vi "Logging Message Loop.vi"(8 "error in (no error)":errorcluster, 10 "Data Queue":refnum<queue>, 11 "Message Queues":T1) -> (0 "error out":errorcluster)   [LabVIEW 2016, in "Logging.lvlib"]
doc: "The message loop subVI to handle messages pertaining to logging data."
uses:
  Logging.lvlib
  support/Message Queue/All Message Queues.ctl
  support/Message Queue/Message Cluster.ctl
  Logging Configuration.ctl
  Logging State.ctl
  support/Message Queue/Enqueue Message (Single).vi
  <vilib>/Utility/error.llb/Error Cluster From Error Code.vi
  <vilib>/ErrorRing/Error Ring.xnode
  support/Message Queue/Message Queue.lvlib
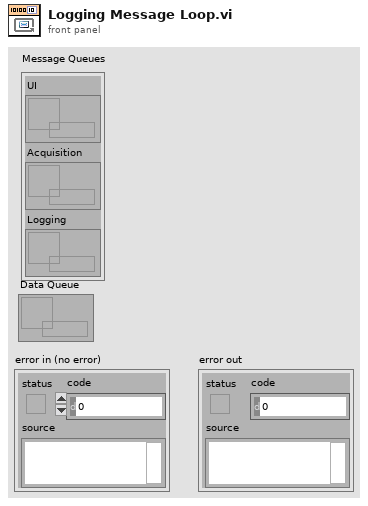
[diagram p1: front panel]
types:
  T1 = typedef "Message Queue.lvlib/All Message Queues.ctl" = cluster{"UI":refnum<queue>, "Acquisition":refnum<queue>, "Logging":refnum<queue>}
  T2 = typedef "Logging.lvlib/Logging Configuration.ctl" = cluster{"Log File Base Path":path, "save file":bool, "refnum out":refnum<file>}
  T3 = enum16{"open", "replace", "create", "open or create", "replace or create", "replace or create with confirmation"}
  T4 = typedef "Logging.lvlib/Logging State.ctl" = enum16{"Idle", "Logging"}
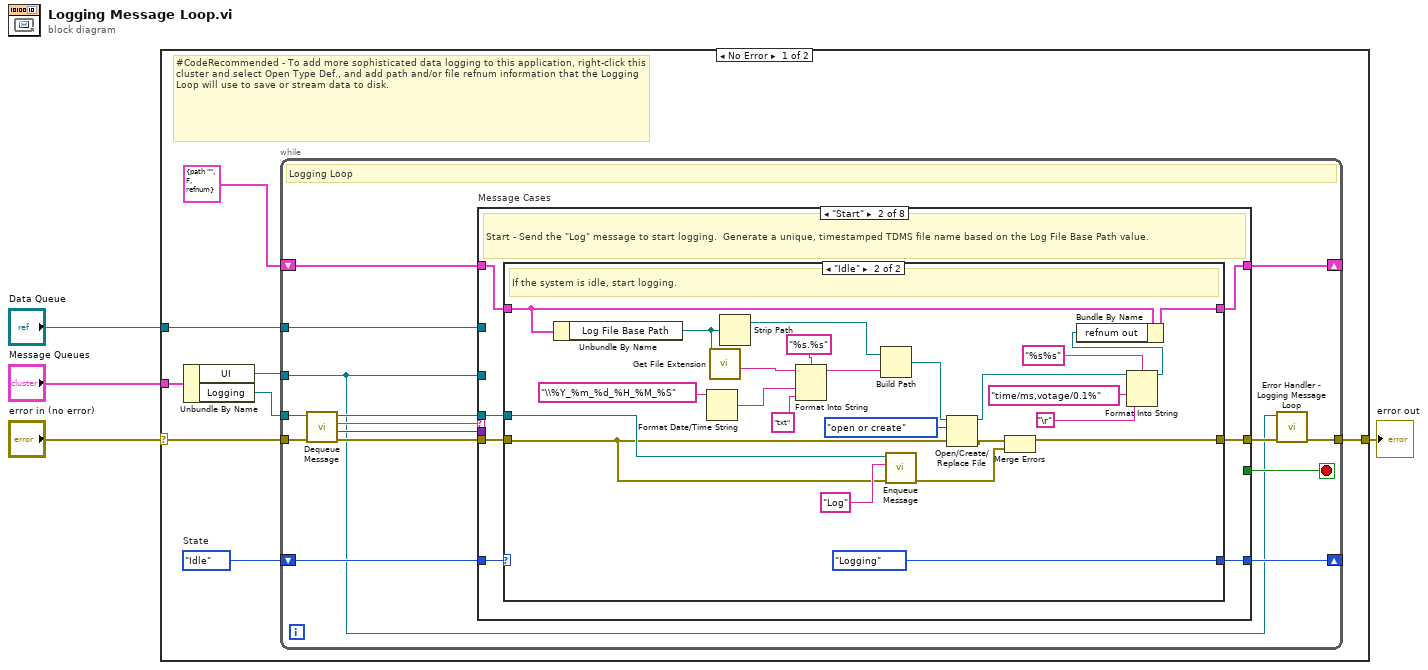
[diagram p0: block diagram]
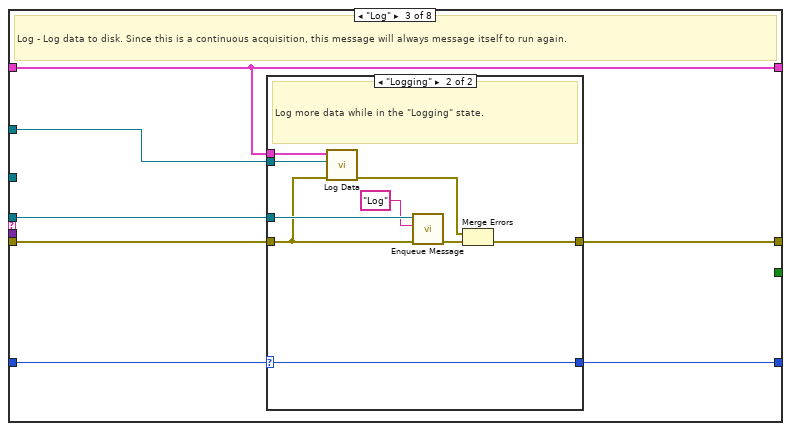
[diagram p4: hidden frame]
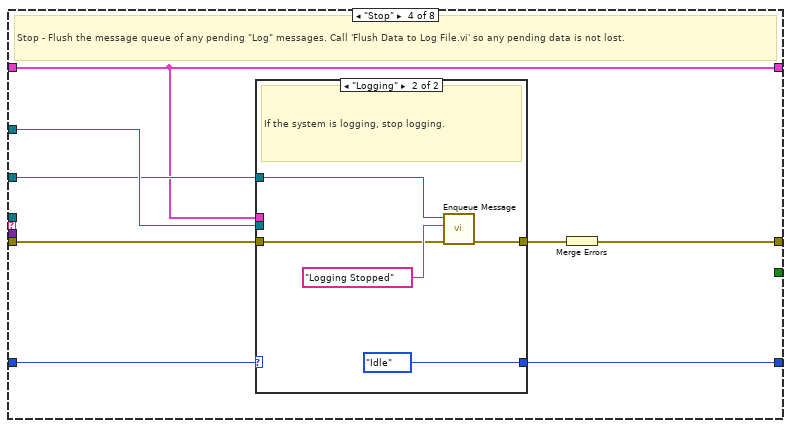
[diagram p6: hidden frame]
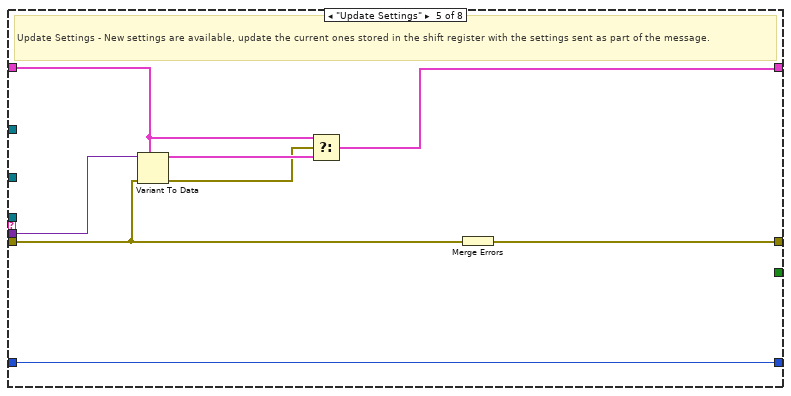
[diagram p8: hidden frame]
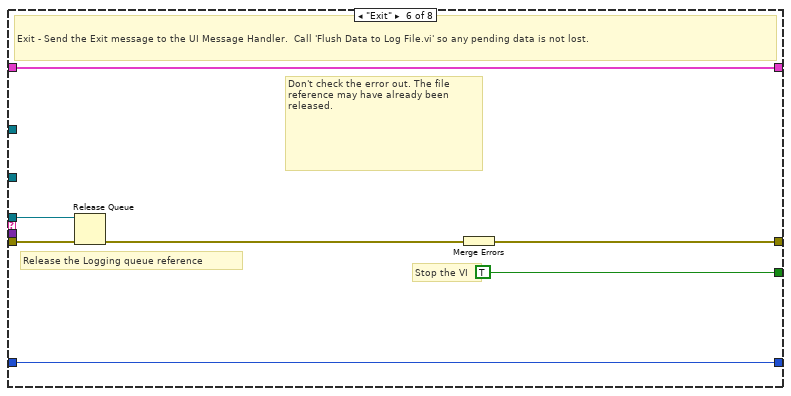
[diagram p9: hidden frame]
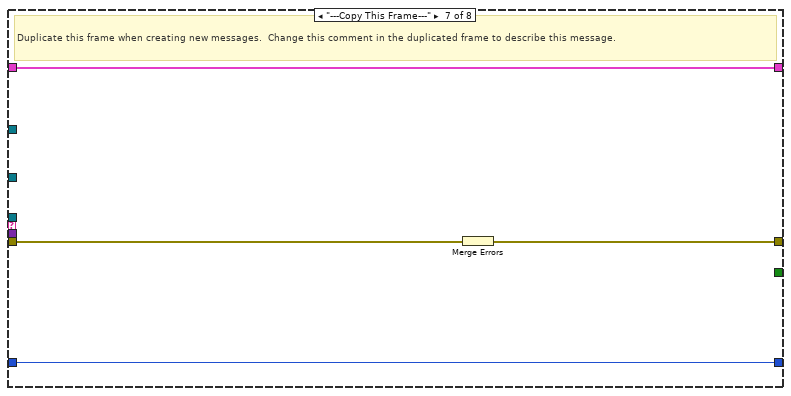
[diagram p10: hidden frame]
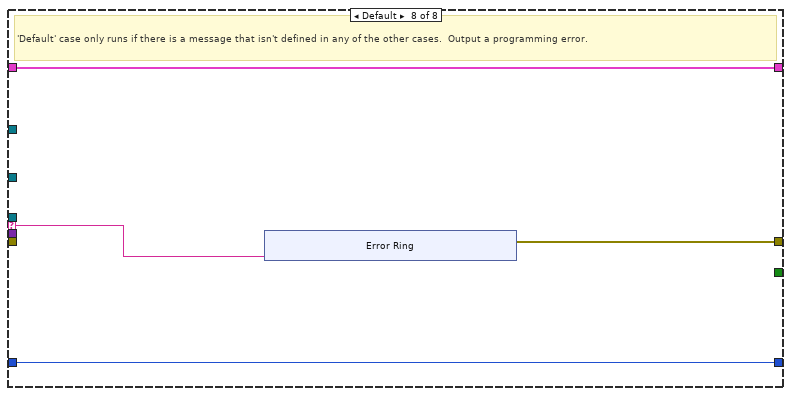
[diagram p11: hidden frame]
diagram:
  n1 = case shown="No Error" "error in (no error)" {
    selector: "error in (no error)" -> [w8 w128]
    tunnel: "Message Queues" -> [w12 _]
    tunnel: [w10 w128] -> w3
    tunnel: "Data Queue" -> [w7 _]
    frame No Error {
      w5 = Logging_State."Idle"  # State
      # "#CodeRecommended - To add more sophisticated data logging to this application, right-click this cluster and select Open Type Def., and add path and/or file refnum information that the Logging Loop will use to save or stream data to disk."
      n2 = Unbundle By Name(w12) -> ("UI"=w6:refnum<queue>, "Logging"=w11:refnum<queue>)
      n3 = while {
        tunnel: w11 -> [w19]
        shift-right: [w26] -> _
        shift-left: T2 {"Log File Base Path"=path "", "save file"=FALSE, "refnum out"=refnum} ("Logging Configuration") -> [w27]
        tunnel: w6 -> [w13]
        tunnel: w7 -> [w18]
        shift-right: [w16] -> _
        shift-left: w5 -> [w17]
        tunnel: w8 -> [w24]
        tunnel: [w15] -> w10
        stop <- w25 stop-if-true
        # "Logging Loop"
        n4 = call "Dequeue Message.vi"("error in (no error)"=w24, "Message Queue"=w19) -> ("error out"=w23:errorcluster, "Message Data"=w21:variant, "Message"=w22:string, "dup Message Queue"=w20:refnum<queue>)  [unwired: 6 in]
        n5 = case "Message Cases" shown="\"Start\"" w22 {
          selector: w22 -> [_ _ _ _ _ _ _ w117]
          tunnel: w20 -> [_ w36 w70 _ _ w109 _ _]
          tunnel: w23 -> [w29 w35 w68 w87 w99 w110 w116 _]
          tunnel: [w29 w37 w71 w90 w105 w111 w114 w118] -> w14
          tunnel: w27 -> [w30 w34 w67 w83 w103 w107 w115 w120]
          tunnel: [w30 w33 w67 w83 w100 w107 w115 w120] -> w26
          tunnel: [_ _ _ _ _ TRUE _ _] -> w25
          tunnel: w21 -> [_ _ _ _ w104 _ _ _]
          tunnel: w13 -> [_ _ _ w84 _ _ _ _]
          tunnel: w18 -> [_ _ w69 w88 _ _ _ _]
          tunnel: w17 -> [w28 w32 w66 w86 w98 w106 w113 w119]
          tunnel: [w28 w31 w65 w85 w98 w106 w113 w119] -> w16
          frame "Initialize" {
            # "Initialize - gets called when first launched. Currently a no-op."
          }
          frame "Start" {
            # "Start - Send the \"Log\" message to start logging.  Generate a unique, timestamped TDMS file name based on the Log File Base Path value."
            n6 = case shown="\"Idle\"" w32 {
              selector: w32 -> [w39 _]
              tunnel: [w38 w51] -> w37
              tunnel: w36 -> [_ w52]
              tunnel: w35 -> [w38 w49]
              tunnel: w34 -> [w40 w53]
              tunnel: [w40 w55] -> w33
              tunnel: [w39 Logging_State."Logging" ("State")] -> w31
              frame "Logging" {
                # "The system is already logging. Ignore the \"Start\" message."
              }
              frame "Idle" {
                # "If the system is idle, start logging."
                n7 = Unbundle By Name(w53) -> ("Log File Base Path"=w63:path)
                n8 = Format Date/Time String(time format string (%c)="\\%Y_%m_%d_%H_%M_%S") -> (date/time string=w58:string)  [unwired: 2 in]
                n9 = call <vilib>:"Get File Extension.vi"("file"=w63) -> ("filename without extension"=w61:string)  [unwired: 6 in, 4 out]
                n10 = Strip Path(path=w63) -> (stripped path=w60:path)  [unwired: 1 out]
                n11 = Format Into String(format string="%s.%s", initial string=w61, w58, "txt" ("input 2")) -> (resulting string=w57:string)  [unwired: 1 in, 1 out]
                n12 = Build Path(base path=w60, name or relative path=w57) -> (appended path=w46:path)
                n13 = call-poly "Enqueue Message.vi"("error in (no error)"=w49, "Message"="Log", "Message Queue"=w52) -> ("error out"=w56:errorcluster)  [unwired: 7 in, 1 out]
                n14 = Open/Create/Replace File(file path (use dialog)=w46, error in=w49, operation (0:open)=T3."open or create") -> (refnum out=w42:refnum<file>, error out=w48:errorcluster)  [unwired: 3 in, 1 out]
                n15 = Merge Errors(w48, w56) -> (w51:errorcluster)
                n16 = Format Into String(format string="%s%s", initial string=w42, "time/ms,votage/0.1%" ("format string"), "\r") -> (resulting string=w41:refnum<file>)  [unwired: 1 in, 1 out]
                n17 = Bundle By Name(cluster=w53, "refnum out"=w41) -> (w55:T2)
              }
            }
          }
          frame "Log" {
            # "Log - Log data to disk. Since this is a continuous acquisition, this message will always message itself to run again."
            n18 = case shown="\"Logging\"" w66 {
              selector: w66 -> [w73 w75]
              tunnel: [w72 w82] -> w71
              tunnel: w70 -> [_ w80]
              tunnel: w69 -> [_ w79]
              tunnel: w68 -> [w72 w74]
              tunnel: w67 -> [_ w76]
              tunnel: [w73 w75] -> w65
              frame "Idle" {
                # "Ignore \"Log\" messages when the logging is idle."
              }
              frame "Logging" {
                # "Log more data while in the \"Logging\" state."
                n19 = call "Log Data.vi"("error in (no error)"=w74, "Data Queue"=w79, "Logging Configuration"=w76) -> ("error out"=w78:errorcluster)  [unwired: 8 in]
                n20 = call-poly "Enqueue Message.vi"("error in (no error)"=w74, "Message"="Log", "Message Queue"=w80) -> ("error out"=w81:errorcluster)  [unwired: 7 in, 1 out]
                n21 = Merge Errors(w78, w81) -> (w82:errorcluster)
              }
            }
          }
          frame "Stop" {
            # "Stop - Flush the message queue of any pending \"Log\" messages. Call 'Flush Data to Log File.vi' so any pending data is not lost."
            n22 = case shown="\"Logging\"" w86 {
              selector: w86 -> [w91 _]
              tunnel: [w92 w96] -> w89
              tunnel: w88 -> [_ _]
              tunnel: w83 -> [_ _]
              tunnel: w87 -> [w92 w93]
              tunnel: [w91 Logging_State."Idle" ("State")] -> w85
              tunnel: w84 -> [_ w95]
              frame "Idle" {
                # "The system is already idle. Ignore the \"Stop\" message."
              }
              frame "Logging" {
                # "If the system is logging, stop logging."
                n23 = call-poly "Enqueue Message.vi"("error in (no error)"=w93, "Message"="Logging Stopped", "Message Queue"=w95) -> ("error out"=w96:errorcluster)  [unwired: 7 in, 1 out]
              }
            }
            n24 = Merge Errors(w89) -> (w90:errorcluster)
          }
          frame "Update Settings" {
            # "Update Settings - New settings are available, update the current ones stored in the shift register with the settings sent as part of the message."
            n25 = Variant To Data(error in=w99, type=w103, Variant=w104) -> (data=w102:T2, error out=w101:errorcluster)
            n26 = Select(t=w103, s=w101, f=w102) -> (s? t:f=w100:T2)
            n27 = Merge Errors(w99) -> (w105:errorcluster)
          }
          frame "Exit" {
            # "Don't check the error out. The file reference may have already been released."
            # "Release the Logging queue reference"
            # "Stop the VI"
            # "Exit - Send the Exit message to the UI Message Handler.  Call 'Flush Data to Log File.vi' so any pending data is not lost."
            n28 = Release Queue(queue=w109, error in (no error)=w110) -> (error out=w108:errorcluster)  [unwired: 1 in, 2 out]
            n29 = Merge Errors(w108) -> (w111:errorcluster)
          }
          frame "---Copy This Frame---" {
            # "Duplicate this frame when creating new messages.  Change this comment in the duplicated frame to describe this message."
            n30 = Merge Errors(w116) -> (w114:errorcluster)
          }
          frame Default {
            # "'Default' case only runs if there is a message that isn't defined in any of the other cases.  Output a programming error."
            n31 = xnode "Error Ring"("parameter 0"=w117) -> ("error out"=w118:errorcluster)
          }
        }
        n32 = call "Error Handler - Logging Message Loop.vi"("error in (no error)"=w14, "Message Queue"=w13) -> ("dup error in"=w15:errorcluster)  [unwired: 8 in, 1 out]
      }
    }
    frame Error {
    }
  }
  "error out" <- w3
